vi "reward.vi"(2 "vars in":T1={"wait count t"=0, "wait min"=0, "wait max"=0, "stim count t"=0, "stim count n"=0, "d stim"=0, "d timeout"=0, "timeout win"=0, "base temp"=0.0, "stim amps"=[], "n hit"=0, "n catch"=0, "active"=TRUE, "catch"=TRUE, "stimulus"=TRUE, "reward given"=TRUE, "pairing"=TRUE, "lick"=FALSE, "next reward"=FALSE, "clean tubes"=FALSE, "next temp"=0.0}) -> (7 "vars out":T1={"wait count t"=0, "wait min"=0, "wait max"=0, "stim count t"=0, "stim count n"=0, "d stim"=0, "d timeout"=0, "timeout win"=0, "base temp"=0.0, "stim amps"=[], "n hit"=0, "n catch"=0, "active"=TRUE, "catch"=TRUE, "stimulus"=TRUE, "reward given"=TRUE, "pairing"=TRUE, "lick"=FALSE, "next reward"=FALSE, "clean tubes"=FALSE, "next temp"=0.0})   [LabVIEW 2015]
uses:
  Type Definitions/vars.ctl
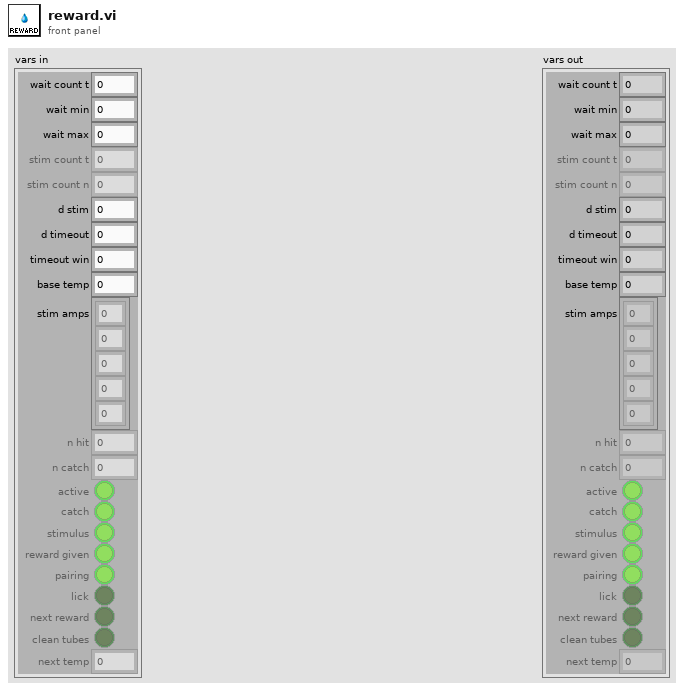
[diagram p1: front panel]
types:
  T1 = typedef "vars.ctl" = cluster{"wait count t":u16, "wait min":u16, "wait max":u16, "stim count t":u16, "stim count n":u16, "d stim":u16, "d timeout":u16, "timeout win":u16, "base temp":sgl, "stim amps":i32[], "n hit":u16, "n catch":u16, "active":bool, "catch":bool, "stimulus":bool, "reward given":bool, "pairing":bool, "lick":bool, "next reward":bool, "clean tubes":bool, "next temp":sgl}
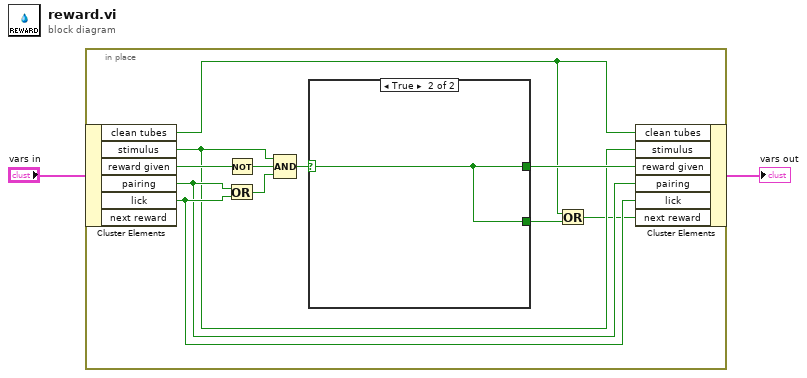
[diagram p0: block diagram]
diagram:
  n1 = in-place {
    n2 = in-place-cluster #1("vars in") -> ("clean tubes"=w3:bool, "stimulus"=w6:bool, "reward given"=w11:bool, "pairing"=w7:bool, "lick"=w8:bool)  [unwired: 1 out]
    n3 = Not(x=w11) -> (.not. x?=w13:bool)
    n4 = Or(x=w7, y=w8) -> (x .or. y?=w12:bool)
    n5 = Compound Arithmetic op=AND(w6, w13, w12) -> (w10:bool)
    n6 = case shown="True" w10 {
      selector: w10 -> [w14 w15]
      tunnel: [w14 w15] -> w9
      tunnel: [w14 w15] -> w5
      frame False {
      }
      frame True {
      }
    }
    n7 = Or(x=w3, y=w5) -> (x .or. y?=w4:bool)
    n8 = in-place-cluster #1("clean tubes"=w3, "stimulus"=w6, "reward given"=w9, "pairing"=w7, "lick"=w8, "next reward"=w4) -> (→"vars out":T1)
  }
